vi "TDMS(Read).vi"(8 "error in (no error)":errorcluster caption="错误输入（无错误）", 11 "文件路径":path) -> (0 "error out":errorcluster caption="错误输出", 2 "通道名称输出":string[](array[string]), 3 "数据":waveform(sgl)[](array[waveform]))   [LabVIEW 2020, in "人体健康监测系统.lvclass"]
uses:
  f905842a-7e08-40ce-9a47-e5fb887419d0.vi
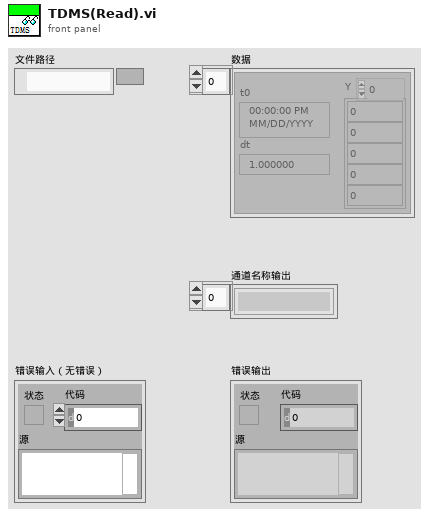
[diagram p1: front panel]
types:
  T1 = enum16{"open", "open or create", "create or replace", "create", "open (read-only)"}
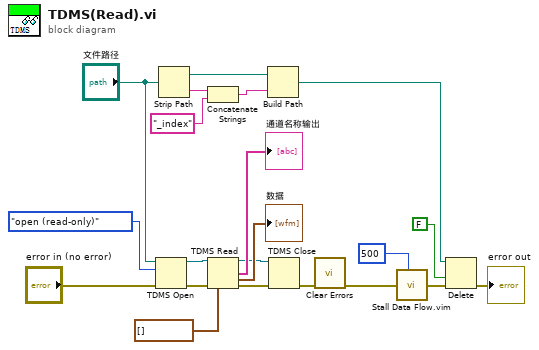
[diagram p0: block diagram]
diagram:
  n1 = TDMS Open(8:"error in (no error)", 10:T1."open (read-only)" ("操作(0:open)"), 11:"文件路径") -> (0:w18:errorcluster, 3:w19:refnum<k34>)  [unwired: 4 in]
  n2 = Strip Path(path="文件路径") -> (stripped path=w8:path, name=w10:string)
  n3 = Concatenate Strings(w10, "_index" ("字符串")) -> (w7:string)
  n4 = TDMS Read(0:w19, 11:w18, 12:waveform(sgl)[] [] ("数据类型")) -> (4:w12:refnum<k34>, 8:→"通道名称输出":string[], 10:→"数据":waveform(sgl)[], 15:w11:errorcluster)  [unwired: 5 in, 2 out]
  n5 = Build Path(base path=w8, name or relative path=w7) -> (appended path=w6:path)
  n6 = TDMS Close(8:w11, 11:w12) -> (0:w17:errorcluster)  [unwired: 1 out]
  n7 = call <vilib>:"Clear Errors.vi"("error in (no error)"=w17) -> ("error out"=w4:errorcluster)  [unwired: 5 in, 1 out]
  n8 = call "Stall Data Flow.vim"("value in"=w4, "milliseconds to wait"=u32 500) -> ("value out"=w3:errorcluster)  [unwired: 1 out]
  n9 = Delete(path (use dialog)=w6, confirm (F)=FALSE ("确认(F)"), error in=w3) -> (error out=→"error out":errorcluster)  [unwired: 2 in, 2 out]
